vi "Register Set Parse.vi"(9 "Register value":u8 format="%.0x", 10 "Register Name":string, 11 "Shadow Reg Ctrls":T1) -> (2 "Cluster Value Array":u32[](array[numeric]), 3 "Cluster Refnum":refnum<vi>)   [LabVIEW 2010]
panel:
  out "array w/ subset deleted":T2(array[cluster])
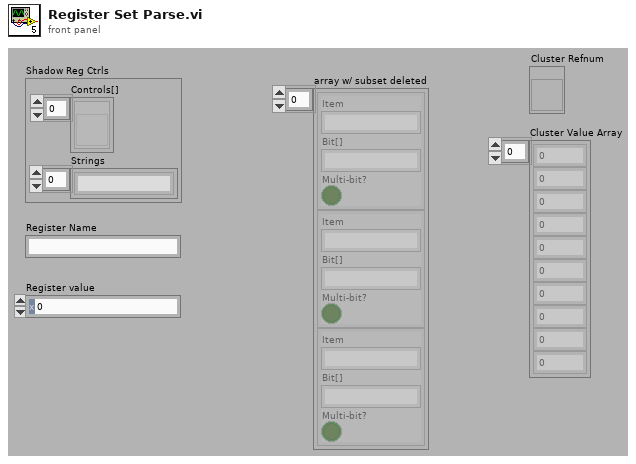
[diagram p1: front panel]
types:
  T1 = cluster{"Controls[]":refnum<vi>[], "Strings":string[]}
  T2 = cluster{"Item":string, "Bit[]":string, "Multi-bit?":bool}[]
  T3 = cluster{"Item":string, "Bit[]":string, "Multi-bit?":bool}
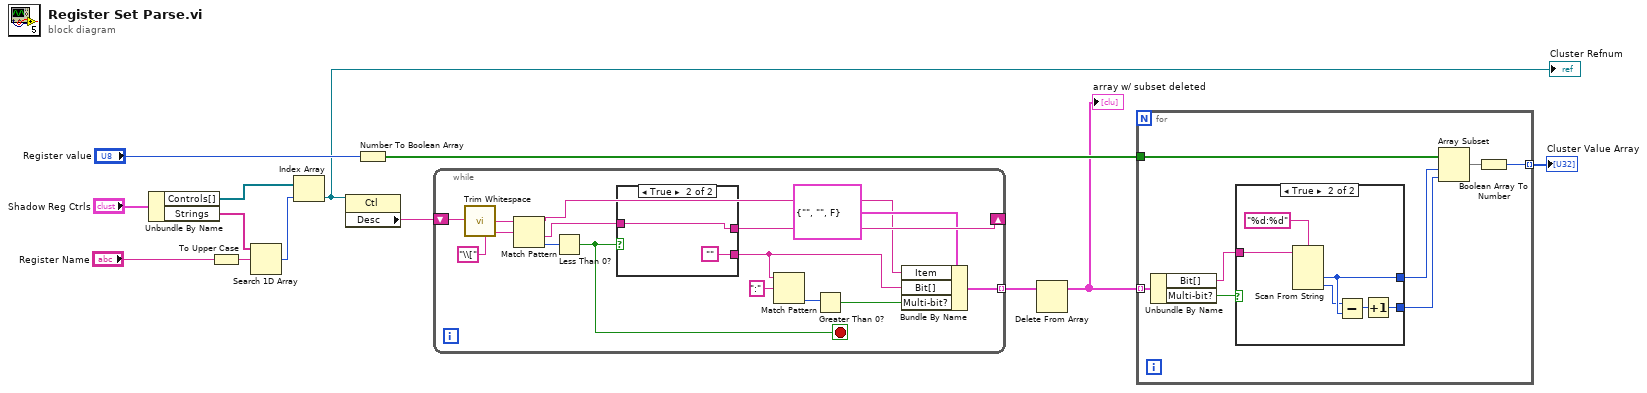
[diagram p0: block diagram]
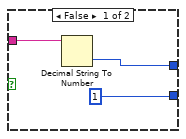
[diagram p2: hidden frame]
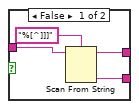
[diagram p3: hidden frame]
diagram:
  n1 = Unbundle By Name("Shadow Reg Ctrls") -> ("Controls[]"=w8:refnum<vi>[], "Strings"=w3:string[])
  n2 = To Upper Case(1:"Register Name") -> (0:w1:string)
  n3 = Search 1D Array(1D array=w3, element=w1) -> (index of element=w6:i32)  [unwired: 1 out]
  n4 = Index Array(array=w8, index=w6) -> (element=w7:refnum<vi>)
  "Cluster Refnum" <- w7
  n5 = property class="Ctl"(reference=w7) -> ("Desc"=w5:string)  [unwired: 1 in, 2 out]
  n6 = Number To Boolean Array(number="Register value") -> (Boolean array=w11:bool[])
  n7 = while {
    shift-right: [w24] -> _
    shift-left: w5 -> [w22]
    tunnel: [w14] -> w12 mode=indexing
    stop <- w25 stop-if-true
    n8 = call <vilib>:"Trim Whitespace.vi"("string"=w22) -> ("trimmed string"=w21:string)  [unwired: 1 in]
    n9 = Match Pattern(string=w21, regular expression="\\[") -> (before substring=w15:string, after substring=w23:string, offset past match=w26:i32)  [unwired: 2 out]
    n10 = Less Than 0?(x=w26) -> (x < 0?=w25:bool)
    n11 = case shown="True" w25 {
      tunnel: w23 -> [w31 w33]
      tunnel: [w29 ""] -> w16
      tunnel: [w28 w33] -> w24
      frame False {
        n12 = Scan From String(format string="%[^]]]", input string=w31) -> (remaining string=w28:string, output 1=w29:string)  [unwired: 2 in, 3 out]
      }
      frame True {
      }
    }
    n13 = Match Pattern(string=w16, regular expression=":") -> (offset past match=w19:i32)  [unwired: 4 out]
    n14 = Greater Than 0?(x=w19) -> (x > 0?=w17:bool)
    n15 = Bundle By Name(cluster=T3 {"Item"="", "Bit[]"="", "Multi-bit?"=FALSE}, "Item"=w15, "Bit[]"=w16, "Multi-bit?"=w17) -> (w14:T3)
  }
  n16 = Delete From Array(array=w12) -> (array with subset deleted=w10:T2)  [unwired: 2 in, 1 out]
  "array w/ subset deleted" <- w10
  n17 = for {
    tunnel: w11 -> [w39]
    tunnel: w10 -> [w41] mode=indexing
    tunnel: [w34] -> w9 mode=indexing
    n18 = Unbundle By Name(w41) -> ("Bit[]"=w38:string, "Multi-bit?"=w40:bool)
    n19 = case shown="True" w40 {
      tunnel: w38 -> [w44 w50]
      tunnel: [w43 w46] -> w37
      tunnel: [1 w48] -> w36
      frame False {
        n20 = Decimal String To Number(string=w44) -> (number=w43:i32)  [unwired: 3 out]
      }
      frame True {
        n21 = Scan From String(format string="%d:%d", input string=w50) -> (output 1=w46:i32, output 2=w45:i32)  [unwired: 2 in, 5 out]
        n22 = Subtract(x=w45, y=w46) -> (x-y=w47:i32)
        n23 = Increment(x=w47) -> (x+1=w48:i32)
      }
    }
    n24 = Array Subset(array=w39, index=w37, length=w36) -> (w35:bool[])
    n25 = Boolean Array To Number(Boolean array=w35) -> (number=w34:u32)
  }
  "Cluster Value Array" <- w9
